vi "Methods_Insert Dividers.vi"(11 "Methods[] In":T1(array[cluster])) -> (3 "Methods[] Out":T1(array[cluster]))   [LabVIEW 2023] (continued)
"Data name"="Statechart.Open Private", "Short name (localized)"="Statechart.Open Private", "Long name (localized)"="Statechart:Open Private"}, "Method Flags"={"IsDeprecated"=FALSE, "IsPrivate"=TRUE, "IsScripting"=FALSE, "IsNotInRun-Time"=FALSE}, "Divider"=FALSE}, {"Class Info"={"Unique ID string"="1", "Parent ID string"="", "Class Name (unlocalized)"="Application", "Class Name (localized)"="Application"}, "Method Info"={"Unique ID string"="90f", "Data name"="Project.DoingAutosaveRecovery", "Short name (localized)"="Project.DoingAutosaveRecovery", "Long name (localized)"="Project:Doing Auto Save Recovery"}, "Method Flags"={"IsDeprecated"=FALSE, "IsPrivate"=TRUE, "IsScripting"=FALSE, "IsNotInRun-Time"=FALSE}, "Divider"=FALSE}, {"Class Info"={"Unique ID string"="1", "Parent ID string"="", "Class Name (unlocalized)"="Application", "Class Name (localized)"="Application"}, "Method Info"={"Unique ID string"="910", "Data name"="AllowScripting", "Short name (localized)"="AllowScripting", "Long name (localized)"="Allow Scripting"}, "Method Flags"={"IsDeprecated"=FALSE, "IsPrivate"=TRUE, "IsScripting"=TRUE, "IsNotInRun-Time"=FALSE}, "Divider"=FALSE}, {"Class Info"={"Unique ID string"="1", "Parent ID string"="", "Class Name (unlocalized)"="Application", "Class Name (localized)"="Application"}, "Method Info"={"Unique ID string"="911", "Data name"="EnableExternalProptypes", "Short name (localized)"="EnableExternalProptypes", "Long name (localized)"="Enable External Proptypes"}, "Method Flags"={"IsDeprecated"=FALSE, "IsPrivate"=TRUE, "IsScripting"=TRUE, "IsNotInRun-Time"=FALSE}, "Divider"=FALSE}, {"Class Info"={"Unique ID string"="1", "Parent ID string"="", "Class Name (unlocalized)"="Application", "Class Name (localized)"="Application"}, "Method Info"={"Unique ID string"="912", "Data name"="EnableTempSelect", "Short name (localized)"="EnableTempSelect", "Long name (localized)"="Enable Temp Selection"}, "Method Flags"={"IsDeprecated"=FALSE, "IsPrivate"=TRUE, "IsScripting"=FALSE, "IsNotInRun-Time"=FALSE}, "Divider"=FALSE}, {"Class Info"={"Unique ID string"="1", "Parent ID string"="", "Class Name (unlocalized)"="Application", "Class Name (localized)"="Application"}, "Method Info"={"Unique ID string"="913", "Data name"="EnableMetaTrans", "Short name (localized)"="EnableMetaTrans", "Long name (localized)"="Enable Meta Transactions"}, "Method Flags"={"IsDeprecated"=FALSE, "IsPrivate"=TRUE, "IsScripting"=TRUE, "IsNotInRun-Time"=FALSE}, "Divider"=FALSE}, {"Class Info"={"Unique ID string"="1", "Parent ID string"="", "Class Name (unlocalized)"="Application", "Class Name (localized)"="Application"}, "Method Info"={"Unique ID string"="914", "Data name"="Symbols.GetValue", "Short name (localized)"="Symbols.GetValue", "Long name (localized)"="Symbols:Get Value"}, "Method Flags"={"IsDeprecated"=FALSE, "IsPrivate"=TRUE, "IsScripting"=FALSE, "IsNotInRun-Time"=TRUE}, "Divider"=FALSE}, {"Class Info"={"Unique ID string"="1", "Parent ID string"="", "Class Name (unlocalized)"="Application", "Class Name (localized)"="Application"}, "Method Info"={"Unique ID string"="915", "Data name"="DeferErrWinUpdates", "Short name (localized)"="DeferErrWinUpdates", "Long name (localized)"="Error Window:Defer Updates"}, "Method Flags"={"IsDeprecated"=FALSE, "IsPrivate"=TRUE, "IsScripting"=FALSE, "IsNotInRun-Time"=TRUE}, "Divider"=FALSE}, {"Class Info"={"Unique ID string"="1", "Parent ID string"="", "Class Name (unlocalized)"="Application", "Class Name (localized)"="Application"}, "Method Info"={"Unique ID string"="916", "Data name"="DTT.IsTracingEnabled", "Short name (localized)"="DTT.IsTracingEnabled", "Long name (localized)"="Desktop Tracing:Is Tracing Enabled"}, "Method Flags"={"IsDeprecated"=FALSE, "IsPrivate"=TRUE, "IsScripting"=FALSE, "IsNotInRun-Time"=FALSE}, "Divider"=FALSE}, {"Class Info"={"Unique ID string"="1", "Parent ID string"="", "Class Name (unlocalized)"="Application", "Class Name (localized)"="Application"}, "Method Info"={"Unique ID string"="917", "Data name"="WebSrvr.Conf", "Short name (localized)"="WebSrvr.Conf", "Long name (localized)"="Web Server:Configure"}, "Method Flags"={"IsDeprecated"=FALSE, "IsPrivate"=FALSE, "IsScripting"=FALSE, "IsNotInRun-Time"=FALSE}, "Divider"=FALSE}, {"Class Info"={"Unique ID string"="1", "Parent ID string"="", "Class Name (unlocalized)"="Application", "Class Name (localized)"="Application"}, "Method Info"={"Unique ID string"="918", "Data name"="CheckMathScriptWatchedPaths", "Short name (localized)"="CheckMathScriptWatchedPaths", "Long name (localized)"="MathScript:Check Watched Paths"}, "Method Flags"={"IsDeprecated"=FALSE, "IsPrivate"=TRUE, "IsScripting"=TRUE, "IsNotInRun-Time"=TRUE}, "Divider"=FALSE}, {"Class Info"={"Unique ID string"="1", "Parent ID string"="", "Class Name (unlocalized)"="Application", "Class Name (localized)"="Application"}, "Method Info"={"Unique ID string"="919", "Data name"="Open.LV Documents", "Short name (localized)"="Open.LV Documents", "Long name (localized)"="Open:LabVIEW Documents"}, "Method Flags"={"IsDeprecated"=FALSE, "IsPrivate"=TRUE, "IsScripting"=FALSE, "IsNotInRun-Time"=TRUE}, "Divider"=FALSE}, {"Class Info"={"Unique ID string"="1", "Parent ID string"="", "Class Name (unlocalized)"="Application", "Class Name (localized)"="Application"}, "Method Info"={"Unique ID string"="91a", "Data name"="Get VI.ConPane DataType", "Short name (localized)"="Get VI.ConPane DataType", "Long name (localized)"="Get VI:ConPane DataType"}, "Method Flags"={"IsDeprecated"=FALSE, "IsPrivate"=FALSE, "IsScripting"=TRUE, "IsNotInRun-Time"=FALSE}, "Divider"=FALSE}, {"Class Info"={"Unique ID string"="1", "Parent ID string"="", "Class Name (unlocalized)"="Application", "Class Name (localized)"="Application"}, "Method Info"={"Unique ID string"="91b", "Data name"="GetActiveVIRef", "Short name (localized)"="GetActiveVIRef", "Long name (localized)"="Get Active VI Reference"}, "Method Flags"={"IsDeprecated"=FALSE, "IsPrivate"=FALSE, "IsScripting"=TRUE, "IsNotInRun-Time"=TRUE}, "Divider"=FALSE}, {"Class Info"={"Unique ID string"="1", "Parent ID string"="", "Class Name (unlocalized)"="Application", "Class Name (localized)"="Application"}, "Method Info"={"Unique ID string"="91c", "Data name"="CodeCov.Start", "Short name (localized)"="CodeCov.Start", "Long name (localized)"="Code Coverage:Start"}, "Method Flags"={"IsDeprecated"=FALSE, "IsPrivate"=TRUE, "IsScripting"=FALSE, "IsNotInRun-Time"=TRUE}, "Divider"=FALSE}, {"Class Info"={"Unique ID string"="1", "Parent ID string"="", "Class Name (unlocalized)"="Application", "Class Name (localized)"="Application"}, "Method Info"={"Unique ID string"="91d", "Data name"="CodeCov.Stop", "Short name (localized)"="CodeCov.Stop", "Long name (localized)"="Code Coverage:Stop"}, "Method Flags"={"IsDeprecated"=FALSE, "IsPrivate"=TRUE, "IsScripting"=FALSE, "IsNotInRun-Time"=TRUE}, "Divider"=FALSE}, {"Class Info"={"Unique ID string"="1", "Parent ID string"="", "Class Name (unlocalized)"="Application", "Class Name (localized)"="Application"}, "Method Info"={"Unique ID string"="91e", "Data name"="CodeCov.Reset", "Short name (localized)"="CodeCov.Reset", "Long name (localized)"="Code Coverage:Reset"}, "Method Flags"={"IsDeprecated"=FALSE, "IsPrivate"=TRUE, "IsScripting"=FALSE, "IsNotInRun-Time"=TRUE}, "Divider"=FALSE}, {"Class Info"={"Unique ID string"="1", "Parent ID string"="", "Class Name (unlocalized)"="Application", "Class Name (localized)"="Application"}, "Method Info"={"Unique ID string"="91f", "Data name"="CodeCov.Reset VI", "Short name (localized)"="CodeCov.Reset VI", "Long name (localized)"="Code Coverage:Reset VI"}, "Method Flags"={"IsDeprecated"=FALSE, "IsPrivate"=TRUE, "IsScripting"=FALSE, "IsNotInRun-Time"=TRUE}, "Divider"=FALSE}, {"Class Info"={"Unique ID string"="1", "Parent ID string"="", "Class Name (unlocalized)"="Application", "Class Name (localized)"="Application"}, "Method Info"={"Unique ID string"="920", "Data name"="CodeCov.AllVIs", "Short name (localized)"="CodeCov.AllVIs", "Long name (localized)"="Code Coverage:All VIs Measured"}, "Method Flags"={"IsDeprecated"=FALSE, "IsPrivate"=TRUE, "IsScripting"=FALSE, "IsNotInRun-Time"=TRUE}, "Divider"=FALSE}, {"Class Info"={"Unique ID string"="1", "Parent ID string"="", "Class Name (unlocalized)"="Application", "Class Name (localized)"="Application"}, "Method Info"={"Unique ID string"="921", "Data name"="CodeCov.VIPercentage", "Short name (localized)"="CodeCov.VIPercentage", "Long name (localized)"="Code Coverage:VI Percentage"}, "Method Flags"={"IsDeprecated"=FALSE, "IsPrivate"=TRUE, "IsScripting"=FALSE, "IsNotInRun-Time"=TRUE}, "Divider"=FALSE}, {"Class Info"={"Unique ID string"="1", "Parent ID string"="", "Class Name (unlocalized)"="Application", "Class Name (localized)"="Application"}, "Method Info"={"Unique ID string"="922", "Data name"="CodeCov.UnrunDiags", "Short name (localized)"="CodeCov.UnrunDiags", "Long name (localized)"="Code Coverage:Uncovered Diagrams"}, "Method Flags"={"IsDeprecated"=FALSE, "IsPrivate"=TRUE, "IsScripting"=FALSE, "IsNotInRun-Time"=TRUE}, "Divider"=FALSE}, {"Class Info"={"Unique ID string"="1", "Parent ID string"="", "Class Name (unlocalized)"="Application", "Class Name (localized)"="Application"}, "Method Info"={"Unique ID string"="923", "Data name"="CodeCov.ShowUnrunDiags", "Short name (localized)"="CodeCov.ShowUnrunDiags", "Long name (localized)"="Code Coverage:Show Uncovered Diagrams"}, "Method Flags"={"IsDeprecated"=FALSE, "IsPrivate"=TRUE, "IsScripting"=FALSE, "IsNotInRun-Time"=TRUE}, "Divider"=FALSE}, {"Class Info"={"Unique ID string"="1", "Parent ID string"="", "Class Name (unlocalized)"="Application", "Class Name (localized)"="Application"}, "Method Info"={"Unique ID string"="924", "Data name"="UI:Abort Merge VIs", "Short name (localized)"="UI:Abort Merge VIs", "Long name (localized)"="User Interaction:Abort Merge VIs"}, "Method Flags"={"IsDeprecated"=FALSE, "IsPrivate"=TRUE, "IsScripting"=FALSE, "IsNotInRun-Time"=TRUE}, "Divider"=FALSE}, {"Class Info"={"Unique ID string"="1", "Parent ID string"="", "Class Name (unlocalized)"="Application", "Class Name (localized)"="Application"}, "Method Info"={"Unique ID string"="925", "Data name"="UI:Merge Load VI", "Short name (localized)"="UI:Merge Load VI", "Long name (localized)"="User Interaction:Merge Load VI"}, "Method Flags"={"IsDeprecated"=FALSE, "IsPrivate"=TRUE, "IsScripting"=FALSE, "IsNotInRun-Time"=TRUE}, "Divider"=FALSE}, {"Class Info"={"Unique ID string"="1", "Parent ID string"="", "Class Name (unlocalized)"="Application", "Class Name (localized)"="Application"}, "Method Info"={"Unique ID string"="926", "Data name"="UI:Merge Save VI", "Short name (localized)"="UI:Merge Save VI", "Long name (localized)"="User Interaction:Merge Save VI"}, "Method Flags"={"IsDeprecated"=FALSE, "IsPrivate"=TRUE, "IsScripting"=FALSE, "IsNotInRun-Time"=TRUE}, "Divider"=FALSE}, {"Class Info"={"Unique ID string"="1", "Parent ID string"="", "Class Name (unlocalized)"="Application", "Class Name (localized)"="Application"}, "Method Info"={"Unique ID string"="927", "Data name"="UI:Merge Cross Load VI", "Short name (localized)"="UI:Merge Cross Load VI", "Long name (localized)"="User Interaction:Merge Cross Load VI"}, "Method Flags"={"IsDeprecated"=FALSE, "IsPrivate"=TRUE, "IsScripting"=FALSE, "IsNotInRun-Time"=TRUE}, "Divider"=FALSE}, {"Class Info"={"Unique ID string"="1", "Parent ID string"="", "Class Name (unlocalized)"="Application", "Class Name (localized)"="Application"}, "Method Info"={"Unique ID string"="928", "Data name"="UI:Merge Close VI", "Short name (localized)"="UI:Merge Close VI", "Long name (localized)"="User Interaction:Merge Close VI"}, "Method Flags"={"IsDeprecated"=FALSE, "IsPrivate"=TRUE, "IsScripting"=FALSE, "IsNotInRun-Time"=TRUE}, "Divider"=FALSE}, {"Class Info"={"Unique ID string"="1", "Parent ID string"="", "Class Name (unlocalized)"="Application", "Class Name (localized)"="Application"}, "Method Info"={"Unique ID string"="929", "Data name"="UI:Merge Load Library", "Short name (localized)"="UI:Merge Load Library", "Long name (localized)"="User Interaction:Merge Load Library"}, "Method Flags"={"IsDeprecated"=FALSE, "IsPrivate"=TRUE, "IsScripting"=FALSE, "IsNotInRun-Time"=TRUE}, "Divider"=FALSE}, {"Class Info"={"Unique ID string"="1", "Parent ID string"="", "Class Name (unlocalized)"="Application", "Class Name (localized)"="Application"}, "Method Info"={"Unique ID string"="92a", "Data name"="UI:Merge Close Library", "Short name (localized)"="UI:Merge Close Library", "Long name (localized)"="User Interaction:Merge Close Library"}, "Method Flags"={"IsDeprecated"=FALSE, "IsPrivate"=TRUE, "IsScripting"=FALSE, "IsNotInRun-Time"=TRUE}, "Divider"=FALSE}, {"Class Info"={"Unique ID string"="1", "Parent ID string"="", "Class Name (unlocalized)"="Application", "Class Name (localized)"="Application"}, "Method Info"={"Unique ID string"="92b", "Data name"="UI:Merge Clean Up Context", "Short name (localized)"="UI:Merge Clean Up Context", "Long name (localized)"="User Interaction:Merge Clean Up Context"}, "Method Flags"={"IsDeprecated"=FALSE, "IsPrivate"=TRUE, "IsScripting"=FALSE, "IsNotInRun-Time"=TRUE}, "Divider"=FALSE}, {"Class Info"={"Unique ID string"="1", "Parent ID string"="", "Class Name (unlocalized)"="Application", "Class Name (localized)"="Application"}, "Method Info"={"Unique ID string"="92c", "Data name"="UI:Merge Save Library", "Short name (localized)"="UI:Merge Save Library", "Long name (localized)"="User Interaction:Merge Save Library"}, "Method Flags"={"IsDeprecated"=FALSE, "IsPrivate"=TRUE, "IsScripting"=FALSE, "IsNotInRun-Time"=TRUE}, "Divider"=FALSE}, {"Class Info"={"Unique ID string"="1", "Parent ID string"="", "Class Name (unlocalized)"="Application", "Class Name (localized)"="Application"}, "Method Info"={"Unique ID string"="92d", "Data name"="License.Get Feature Activators", "Short name (localized)"="License.Get Feature Activators", "Long name (localized)"="License:Get Feature Activators"}, "Method Flags"={"IsDeprecated"=FALSE, "IsPrivate"=TRUE, "IsScripting"=FALSE, "IsNotInRun-Time"=FALSE}, "Divider"=FALSE}, {"Class Info"={"Unique ID string"="1", "Parent ID string"="", "Class Name (unlocalized)"="Application", "Class Name (localized)"="Application"}, "Method Info"={"Unique ID string"="92e", "Data name"="UI:Merge Load Refees", "Short name (localized)"="UI:Merge Load Refees", "Long name (localized)"="User Interaction:Merge Load Refees"}, "Method Flags"={"IsDeprecated"=FALSE, "IsPrivate"=TRUE, "IsScripting"=FALSE, "IsNotInRun-Time"=TRUE}, "Divider"=FALSE}, {"Class Info"={"Unique ID string"="1", "Parent ID string"="", "Class Name (unlocalized)"="Application", "Class Name (localized)"="Application"}, "Method Info"={"Unique ID string"="92f", "Data name"="Library.Undeploy Libraries", "Short name (localized)"="Library.Undeploy Libraries", "Long name (localized)"="Library:Undeploy Libraries"}, "Method Flags"={"IsDeprecated"=FALSE, "IsPrivate"=FALSE, "IsScripting"=FALSE, "IsNotInRun-Time"=FALSE}, "Divider"=FALSE}, {"Class Info"={"Unique ID string"="1", "Parent ID string"="", "Class Name (unlocalized)"="Application", "Class Name (localized)"="Application"}, "Method Info"={"Unique ID string"="930", "Data name"="Close All Palettes", "Short name (localized)"="Close All Palettes", "Long name (localized)"="Palettes:Close All Palettes"}, "Method Flags"={"IsDeprecated"=FALSE, "IsPrivate"=FALSE, "IsScripting"=FALSE, "IsNotInRun-Time"=TRUE}, "Divider"=FALSE}, {"Class Info"={"Unique ID string"="1", "Parent ID string"="", "Class Name (unlocalized)"="Application", "Class Name (localized)"="Application"}, "Method Info"={"Unique ID string"="931", "Data name"="UI.Edit Icon", "Short name (localized)"="UI.Edit Icon", "Long name (localized)"="User Interaction:Edit Icon"}, "Method Flags"={"IsDeprecated"=FALSE, "IsPrivate"=TRUE, "IsScripting"=FALSE, "IsNotInRun-Time"=TRUE}, "Divider"=FALSE}, {"Class Info"={"Unique ID string"="1", "Parent ID string"="", "Class Name (unlocalized)"="Application", "Class Name (localized)"="Application"}, "Method Info"={"Unique ID string"="932", "Data name"="CreateInstantiation", "Short name (localized)"="CreateInstantiation", "Long name (localized)"="Create Generic VI Instantiation"}, "Method Flags"={"IsDeprecated"=FALSE, "IsPrivate"=TRUE, "IsScripting"=TRUE, "IsNotInRun-Time"=TRUE}, "Divider"=FALSE}, {"Class Info"={"Unique ID string"="1", "Parent ID string"="", "Class Name (unlocalized)"="Application", "Class Name (localized)"="Application"}, "Method Info"={"Unique ID string"="933", "Data name"="Move VIs", "Short name (localized)"="Move VIs", "Long name (localized)"="Move VIs"}, "Method Flags"={"IsDeprecated"=FALSE, "IsPrivate"=TRUE, "IsScripting"=FALSE, "IsNotInRun-Time"=FALSE}, "Divider"=FALSE}, {"Class Info"={"Unique ID string"="1", "Parent ID string"="", "Class Name (unlocalized)"="Application", "Class Name (localized)"="Application"}, "Method Info"={"Unique ID string"="935", "Data name"="Library.Get Ref By Qualified Name", "Short name (localized)"="Library.Get Ref By Qualified Name", "Long name (localized)"="Library:Get Ref By Qualified Name"}, "Method Flags"={"IsDeprecated"=FALSE, "IsPrivate"=FALSE, "IsScripting"=FALSE, "IsNotInRun-Time"=FALSE}, "Divider"=FALSE}, {"Class Info"={"Unique ID string"="1", "Parent ID string"="", "Class Name (unlocalized)"="Application", "Class Name (localized)"="Application"}, "Method Info"={"Unique ID string"="936", "Data name"="CopyDataConvert", "Short name (localized)"="CopyDataConvert", "Long name (localized)"="Copy Data Convert"}, "Method Flags"={"IsDeprecated"=FALSE, "IsPrivate"=TRUE, "IsScripting"=TRUE, "IsNotInRun-Time"=FALSE}, "Divider"=FALSE}, {"Class Info"={"Unique ID string"="1", "Parent ID string"="", "Class Name (unlocalized)"="Application", "Class Name (localized)"="Application"}, "Method Info"={"Unique ID string"="937", "Data name"="LoadMSCompiler", "Short name (localized)"="LoadMSCompiler", "Long name (localized)"="MathScript:Load MathScript Compiler"}, "Method Flags"={"IsDeprecated"=FALSE, "IsPrivate"=TRUE, "IsScripting"=FALSE, "IsNotInRun-Time"=TRUE}, "Divider"=FALSE}, {"Class Info"={"Unique ID string"="1", "Parent ID string"="", "Class Name (unlocalized)"="Application", "Class Name (localized)"="Application"}, "Method Info"={"Unique ID string"="938", "Data name"="Get Hier Img Scaled", "Short name (localized)"="Get Hier Img Scaled", "Long name (localized)"="Get VI Hierarchy Image Scaled"}, "Method Flags"={"IsDeprecated"=FALSE, "IsPrivate"=FALSE, "IsScripting"=FALSE, "IsNotInRun-Time"=FALSE}, "Divider"=FALSE}, {"Class Info"={"Unique ID string"="1", "Parent ID string"="", "Class Name (unlocalized)"="Application", "Class Name (localized)"="Application"}, "Method Info"={"Unique ID string"="939", "Data name"="SearchOpenSession", "Short name (localized)"="SearchOpenSession", "Long name (localized)"="Search:Open Session"}, "Method Flags"={"IsDeprecated"=FALSE, "IsPrivate"=TRUE, "IsScripting"=FALSE, "IsNotInRun-Time"=TRUE}, "Divider"=FALSE}, {"Class Info"={"Unique ID string"="1", "Parent ID string"="", "Class Name (unlocalized)"="Application", "Class Name (localized)"="Application"}, "Method Info"={"Unique ID string"="93a", "Data name"="SearchCloseSession", "Short name (localized)"="SearchCloseSession", "Long name (localized)"="Search:Close Session"}, "Method Flags"={"IsDeprecated"=FALSE, "IsPrivate"=TRUE, "IsScripting"=FALSE, "IsNotInRun-Time"=TRUE}, "Divider"=FALSE}, {"Class Info"={"Unique ID string"="1", "Parent ID string"="", "Class Name (unlocalized)"="Application", "Class Name (localized)"="Application"}, "Method Info"={"Unique ID string"="93b", "Data name"="SearchLoadPlugin", "Short name (localized)"="SearchLoadPlugin", "Long name (localized)"="Search:Load Plugin"}, "Method Flags"={"IsDeprecated"=FALSE, "IsPrivate"=TRUE, "IsScripting"=FALSE, "IsNotInRun-Time"=TRUE}, "Divider"=FALSE}, {"Class Info"={"Unique ID string"="1", "Parent ID string"="", "Class Name (unlocalized)"="Application", "Class Name (localized)"="Application"}, "Method Info"={"Unique ID string"="93c", "Data name"="SearchInitSession", "Short name (localized)"="SearchInitSession", "Long name (localized)"="Search:Init Session"}, "Method Flags"={"IsDeprecated"=FALSE, "IsPrivate"=TRUE, "IsScripting"=FALSE, "IsNotInRun-Time"=TRUE}, "Divider"=FALSE}, {"Class Info"={"Unique ID string"="1", "Parent ID string"="", "Class Name (unlocalized)"="Application", "Class Name (localized)"="Application"}, "Method Info"={"Unique ID string"="93d", "Data name"="SearchSyncSearch", "Short name (localized)"="SearchSyncSearch", "Long name (localized)"="Search:SyncSearch"}, "Method Flags"={"IsDeprecated"=FALSE, "IsPrivate"=TRUE, "IsScripting"=FALSE, "IsNotInRun-Time"=TRUE}, "Divider"=FALSE}, {"Class Info"={"Unique ID string"="1", "Parent ID string"="", "Class Name (unlocalized)"="Application", "Class Name (localized)"="Application"}, "Method Info"={"Unique ID string"="93e", "Data name"="SearchSyncSearchForQD", "Short name (localized)"="SearchSyncSearchForQD", "Long name (localized)"="Search:Sync Search For QD"}, "Method Flags"={"IsDeprecated"=FALSE, "IsPrivate"=TRUE, "IsScripting"=FALSE, "IsNotInRun-Time"=TRUE}, "Divider"=FALSE}, {"Class Info"={"Unique ID string"="1", "Parent ID string"="", "Class Name (unlocalized)"="Application", "Class Name (localized)"="Application"}, "Method Info"={"Unique ID string"="93f", "Data name"="UI.PlaceObjectOnCursor", "Short name (localized)"="UI.PlaceObjectOnCursor", "Long name (localized)"="User Interaction:Place Object On Cursor"}, "Method Flags"={"IsDeprecated"=FALSE, "IsPrivate"=FALSE, "IsScripting"=TRUE, "IsNotInRun-Time"=TRUE}, "Divider"=FALSE}, {"Class Info"={"Unique ID string"="1", "Parent ID string"="", "Class Name (unlocalized)"="Application", "Class Name (localized)"="Application"}, "Method Info"={"Unique ID string"="940", "Data name"="UI.Drop Proj Item Copy", "Short name (localized)"="UI.Drop Proj Item Copy", "Long name (localized)"="User Interaction:Place Project Item On Cursor"}, "Method Flags"={"IsDeprecated"=FALSE, "IsPrivate"=TRUE, "IsScripting"=FALSE, "IsNotInRun-Time"=TRUE}, "Divider"=FALSE}, {"Class Info"={"Unique ID string"="1", "Parent ID string"="", "Class Name (unlocalized)"="Application", "Class Name (localized)"="Application"}, "Method Info"={"Unique ID string"="941", "Data name"="UpdateNXTContextName", "Short name (localized)"="UpdateNXTContextName", "Long name (localized)"="NXT:Update Context Name"}, "Method Flags"={"IsDeprecated"=FALSE, "IsPrivate"=TRUE, "IsScripting"=FALSE, "IsNotInRun-Time"=TRUE}, "Divider"=FALSE}, {"Class Info"={"Unique ID string"="1", "Parent ID string"="", "Class Name (unlocalized)"="Application", "Class Name (localized)"="Application"}, "Method Info"={"Unique ID string"="942", "Data name"="ClearInstantiationCacheCache", "Short name (localized)"="ClearInstantiationCacheCache", "Long name (localized)"="Clear Instantiation Cache Cache"}, "Method Flags"={"IsDeprecated"=FALSE, "IsPrivate"=TRUE, "IsScripting"=FALSE, "IsNotInRun-Time"=TRUE}, "Divider"=FALSE}, {"Class Info"={"Unique ID string"="1", "Parent ID string"="", "Class Name (unlocalized)"="Application", "Class Name (localized)"="Application"}, "Method Info"={"Unique ID string"="943", "Data name"="GetInstantiationConPaneFromCache", "Short name (localized)"="GetInstantiationConPaneFromCache", "Long name (localized)"="Get Instantiation ConPane From Cache"}, "Method Flags"={"IsDeprecated"=FALSE, "IsPrivate"=TRUE, "IsScripting"=FALSE, "IsNotInRun-Time"=TRUE}, "Divider"=FALSE}, {"Class Info"={"Unique ID string"="1", "Parent ID string"="", "Class Name (unlocalized)"="Application", "Class Name (localized)"="Application"}, "Method Info"={"Unique ID string"="944", "Data name"="DTT.FilterVILibEvents", "Short name (localized)"="DTT.FilterVILibEvents", "Long name (localized)"="Desktop Tracing:Filter VI Lib Events"}, "Method Flags"={"IsDeprecated"=FALSE, "IsPrivate"=TRUE, "IsScripting"=FALSE, "IsNotInRun-Time"=FALSE}, "Divider"=FALSE}, {"Class Info"={"Unique ID string"="1", "Parent ID string"="", "Class Name (unlocalized)"="Application", "Class Name (localized)"="Application"}, "Method Info"={"Unique ID string"="945", "Data name"="LocateMSTargetSyntaxVI", "Short name (localized)"="LocateMSTargetSyntaxVI", "Long name (localized)"="MathScript:Locate Math Script Target Syntax VI"}, "Method Flags"={"IsDeprecated"=FALSE, "IsPrivate"=TRUE, "IsScripting"=FALSE, "IsNotInRun-Time"=TRUE}, "Divider"=FALSE}, {"Class Info"={"Unique ID string"="1", "Parent ID string"="", "Class Name (unlocalized)"="Application", "Class Name (localized)"="Application"}, "Method Info"={"Unique ID string"="946", "Data name"="GetEnvModePath", "Short name (localized)"="GetEnvModePath", "Long name (localized)"="Get Environment Mode Settings Path"}, "Method Flags"={"IsDeprecated"=FALSE, "IsPrivate"=TRUE, "IsScripting"=FALSE, "IsNotInRun-Time"=TRUE}, "Divider"=FALSE}, {"Class Info"={"Unique ID string"="1", "Parent ID string"="", "Class Name (unlocalized)"="Application", "Class Name (localized)"="Application"}, "Method Info"={"Unique ID string"="947", "Data name"="Get VI Editor Version", "Short name (localized)"="Get VI Editor Version", "Long name (localized)"="Get VI:Editor Version"}, "Method Flags"={"IsDeprecated"=FALSE, "IsPrivate"=FALSE, "IsScripting"=FALSE, "IsNotInRun-Time"=FALSE}, "Divider"=FALSE}, {"Class Info"={"Unique ID string"="1", "Parent ID string"="", "Class Name (unlocalized)"="Application", "Class Name (localized)"="Application"}, "Method Info"={"Unique ID string"="948", "Data name"="Get VI.Qualified Name", "Short name (localized)"="Get VI.Qualified Name", "Long name (localized)"="Get VI:Qualified Name"}, "Method Flags"={"IsDeprecated"=FALSE, "IsPrivate"=FALSE, "IsScripting"=FALSE, "IsNotInRun-Time"=FALSE}, "Divider"=FALSE}, {"Class Info"={"Unique ID string"="1", "Parent ID string"="", "Class Name (unlocalized)"="Application", "Class Name (localized)"="Application"}, "Method Info"={"Unique ID string"="949", "Data name"="OpenVIInNXTContext", "Short name (localized)"="OpenVIInNXTContext", "Long name (localized)"="NXT:Open VI In Context"}, "Method Flags"={"IsDeprecated"=FALSE, "IsPrivate"=TRUE, "IsScripting"=FALSE, "IsNotInRun-Time"=TRUE}, "Divider"=FALSE}, {"Class Info"={"Unique ID string"="1", "Parent ID string"="", "Class Name (unlocalized)"="Application", "Class Name (localized)"="Application"}, "Method Info"={"Unique ID string"="94b", "Data name"="App.PrepareToLoadFiles", "Short name (localized)"="App.PrepareToLoadFiles", "Long name (localized)"="Prepare to Load Files"}, "Method Flags"={"IsDeprecated"=FALSE, "IsPrivate"=TRUE, "IsScripting"=FALSE, "IsNotInRun-Time"=FALSE}, "Divider"=FALSE}, {"Class Info"={"Unique ID string"="1", "Parent ID string"="", "Class Name (unlocalized)"="Application", "Class Name (localized)"="Application"}, "Method Info"={"Unique ID string"="94c", "Data name"="Get Pal Item Icon", "Short name (localized)"="Get Pal Item Icon", "Long name (localized)"="Palettes:Get Palette Item Icon"}, "Method Flags"={"IsDeprecated"=FALSE, "IsPrivate"=TRUE, "IsScripting"=FALSE, "IsNotInRun-Time"=TRUE}, "Divider"=FALSE}, {"Class Info"={"Unique ID string"="1", "Parent ID string"="", "Class Name (unlocalized)"="Application", "Class Name (localized)"="Application"}, "Method Info"={"Unique ID string"="94d", "Data name"="ReadDFIRTokens", "Short name (localized)"="ReadDFIRTokens", "Long name (localized)"="Compiler:Read DFIR Tokens"}, "Method Flags"={"IsDeprecated"=FALSE, "IsPrivate"=TRUE, "IsScripting"=FALSE, "IsNotInRun-Time"=FALSE}, "Divider"=FALSE}, {"Class Info"={"Unique ID string"="1", "Parent ID string"="", "Class Name (unlocalized)"="Application", "Class Name (localized)"="Application"}, "Method Info"={"Unique ID string"="94e", "Data name"="CreateProbeVIFromVariant", "Short name (localized)"="CreateProbeVIFromVariant", "Long name (localized)"="Probes:Create Probe VI From Variant"}, "Method Flags"={"IsDeprecated"=FALSE, "IsPrivate"=TRUE, "IsScripting"=TRUE, "IsNotInRun-Time"=TRUE}, "Divider"=FALSE}, {"Class Info"={"Unique ID string"="1", "Parent ID string"="", "Class Name (unlocalized)"="Application", "Class Name (localized)"="Application"}, "Method Info"={"Unique ID string"="94f", "Data name"="GetProbePathListFromVariant", "Short name (localized)"="GetProbePathListFromVariant", "Long name (localized)"="Probes:Get Probe Path List From Variant"}, "Method Flags"={"IsDeprecated"=FALSE, "IsPrivate"=TRUE, "IsScripting"=TRUE, "IsNotInRun-Time"=TRUE}, "Divider"=FALSE}, {"Class Info"={"Unique ID string"="1", "Parent ID string"="", "Class Name (unlocalized)"="Application", "Class Name (localized)"="Application"}, "Method Info"={"Unique ID string"="951", "Data name"="Build.PackedLibrary", "Short name (localized)"="Build.PackedLibrary", "Long name (localized)"="Build:PackedLibrary"}, "Method Flags"={"IsDeprecated"=FALSE, "IsPrivate"=TRUE, "IsScripting"=FALSE, "IsNotInRun-Time"=TRUE}, "Divider"=FALSE}, {"Class Info"={"Unique ID string"="1", "Parent ID string"="", "Class Name (unlocalized)"="Application", "Class Name (localized)"="Application"}, "Method Info"={"Unique ID string"="952", "Data name"="GetCompilerSettings", "Short name (localized)"="GetCompilerSettings", "Long name (localized)"="Compiler:Get Compiler Settings"}, "Method Flags"={"IsDeprecated"=FALSE, "IsPrivate"=TRUE, "IsScripting"=FALSE, "IsNotInRun-Time"=FALSE}, "Divider"=FALSE}, {"Class Info"={"Unique ID string"="1", "Parent ID string"="", "Class Name (unlocalized)"="Application", "Class Name (localized)"="Application"}, "Method Info"={"Unique ID string"="953", "Data name"="SetCompilerSettings", "Short name (localized)"="SetCompilerSettings", "Long name (localized)"="Compiler:Set Compiler Settings"}, "Method Flags"={"IsDeprecated"=FALSE, "IsPrivate"=TRUE, "IsScripting"=FALSE, "IsNotInRun-Time"=FALSE}, "Divider"=FALSE}, {"Class Info"={"Unique ID string"="1", "Parent ID string"="", "Class Name (unlocalized)"="Application", "Class Name (localized)"="Application"}, "Method Info"={"Unique ID string"="954", "Data name"="Project.GetFileLVVersion", "Short name (localized)"="Project.GetFileLVVersion", "Long name (localized)"="Project:Get File LabVIEW Version"}, "Method Flags"={"IsDeprecated"=FALSE, "IsPrivate"=FALSE, "IsScripting"=FALSE, "IsNotInRun-Time"=FALSE}, "Divider"=FALSE}, {"Class Info"={"Unique ID string"="1", "Parent ID string"="", "Class Name (unlocalized)"="Application", "Class Name (localized)"="Application"}, "Method Info"={"Unique ID string"="955", "Data name"="Save All", "Short name (localized)"="Save All", "Long name (localized)"="Save All"}, "Method Flags"={"IsDeprecated"=FALSE, "IsPrivate"=TRUE, "IsScripting"=FALSE, "IsNotInRun-Time"=FALSE}, "Divider"=FALSE}, {"Class Info"={"Unique ID string"="1", "Parent ID string"="", "Class Name (unlocalized)"="Application", "Class Name (localized)"="Application"}, "Method Info"={"Unique ID string"="956", "Data name"="Release LV Class Cookies", "Short name (localized)"="Release LV Class Cookies", "Long name (localized)"="LabVIEW Class:Release LV Class Cookies"}, "Method Flags"={"IsDeprecated"=FALSE, "IsPrivate"=TRUE, "IsScripting"=FALSE, "IsNotInRun-Time"=FALSE}, "Divider"=FALSE}, {"Class Info"={"Unique ID string"="1", "Parent ID string"="", "Class Name (unlocalized)"="Application", "Class Name (localized)"="Application"}, "Method Info"={"Unique ID string"="957", "Data name"="Consolidated Save", "Short name (localized)"="Consolidated Save", "Long name (localized)"="Consolidated Save"}, "Method Flags"={"IsDeprecated"=FALSE, "IsPrivate"=TRUE, "IsScripting"=FALSE, "IsNotInRun-Time"=TRUE}, "Divider"=FALSE}, {"Class Info"={"Unique ID string"="1", "Parent ID string"="", "Class Name (unlocalized)"="Application", "Class Name (localized)"="Application"}, "Method Info"={"Unique ID string"="958", "Data name"="Compare CPTMs For Packed Library", "Short name (localized)"="Compare CPTMs For Packed Library", "Long name (localized)"="Compare:CPTMs For Packed Library"}, "Method Flags"={"IsDeprecated"=FALSE, "IsPrivate"=TRUE, "IsScripting"=FALSE, "IsNotInRun-Time"=FALSE}, "Divider"=FALSE}, {"Class Info"={"Unique ID string"="1", "Parent ID string"="", "Class Name (unlocalized)"="Application", "Class Name (localized)"="Application"}, "Method Info"={"Unique ID string"="959", "Data name"="Get Pal Item Path", "Short name (localized)"="Get Pal Item Path", "Long name (localized)"="Palettes:Get Palette Item Path"}, "Method Flags"={"IsDeprecated"=FALSE, "IsPrivate"=FALSE, "IsScripting"=FALSE, "IsNotInRun-Time"=FALSE}, "Divider"=FALSE}, {"Class Info"={"Unique ID string"="1", "Parent ID string"="", "Class Name (unlocalized)"="Application", "Class Name (localized)"="Application"}, "Method Info"={"Unique ID string"="95a", "Data name"="GetEnvModeDisplayName", "Short name (localized)"="GetEnvModeDisplayName", "Long name (localized)"="Get Environment Mode Display Name"}, "Method Flags"={"IsDeprecated"=FALSE, "IsPrivate"=FALSE, "IsScripting"=FALSE, "IsNotInRun-Time"=FALSE}, "Divider"=FALSE}, {"Class Info"={"Unique ID string"="1", "Parent ID string"="", "Class Name (unlocalized)"="Application", "Class Name (localized)"="Application"}, "Method Info"={"Unique ID string"="95b", "Data name"="ClearCompObjCache", "Short name (localized)"="ClearCompObjCache", "Long name (localized)"="Clear Compiled Object Cache"}, "Method Flags"={"IsDeprecated"=FALSE, "IsPrivate"=FALSE, "IsScripting"=FALSE, "IsNotInRun-Time"=TRUE}, "Divider"=FALSE}, {"Class Info"={"Unique ID string"="1", "Parent ID string"="", "Class Name (unlocalized)"="Application", "Class Name (localized)"="Application"}, "Method Info"={"Unique ID string"="95c", "Data name"="Packed Library.Get Exported File List", "Short name (localized)"="Packed Library.Get Exported File List", "Long name (localized)"="Packed Library:Get Exported File List"}, "Method Flags"={"IsDeprecated"=FALSE, "IsPrivate"=TRUE, "IsScripting"=FALSE, "IsNotInRun-Time"=FALSE}, "Divider"=FALSE}, {"Class Info"={"Unique ID string"="1", "Parent ID string"="", "Class Name (unlocalized)"="Application", "Class Name (localized)"="Application"}, "Method Info"={"Unique ID string"="95d", "Data name"="Library.IsOpenedInAnyContext", "Short name (localized)"="Library.IsOpenedInAnyContext", "Long name (localized)"="Library:Is Opened In Any Context"}, "Method Flags"={"IsDeprecated"=FALSE, "IsPrivate"=TRUE, "IsScripting"=FALSE, "IsNotInRun-Time"=TRUE}, "Divider"=FALSE}, {"Class Info"={"Unique ID string"="1", "Parent ID string"="", "Class Name (unlocalized)"="Application", "Class Name (localized)"="Application"}, "Method Info"={"Unique ID string"="95e", "Data name"="Compile App Context", "Short name (localized)"="Compile App Context", "Long name (localized)"="Compiler:Compile App Context"}, "Method Flags"={"IsDeprecated"=FALSE, "IsPrivate"=TRUE, "IsScripting"=FALSE, "IsNotInRun-Time"=FALSE}, "Divider"=FALSE}, {"Class Info"={"Unique ID string"="1", "Parent ID string"="", "Class Name (unlocalized)"="Application", "Class Name (localized)"="Application"}, "Method Info"={"Unique ID string"="95f", "Data name"="Packed Library.Enable Caching", "Short name (localized)"="Packed Library.Enable Caching", "Long name (localized)"="Packed Library:Enable Caching"}, "Method Flags"={"IsDeprecated"=FALSE, "IsPrivate"=TRUE, "IsScripting"=FALSE, "IsNotInRun-Time"=FALSE}, "Divider"=FALSE}, {"Class Info"={"Unique ID string"="1", "Parent ID string"="", "Class Name (unlocalized)"="Application", "Class Name (localized)"="Application"}, "Method Info"={"Unique ID string"="960", "Data name"="Simulation.GetParamOffsets", "Short name (localized)"="Simulation.GetParamOffsets", "Long name (localized)"="Simulation:Get Parameter Offsets"}, "Method Flags"={"IsDeprecated"=FALSE, "IsPrivate"=TRUE, "IsScripting"=FALSE, "IsNotInRun-Time"=FALSE}, "Divider"=FALSE}, {"Class Info"={"Unique ID string"="1", "Parent ID string"="", "Class Name (unlocalized)"="Application", "Class Name (localized)"="Application"}, "Method Info"={"Unique ID string"="961", "Data name"="LVRT.Get LibP Sigs", "Short name (localized)"="LVRT.Get LibP Sigs", "Long name (localized)"="LVRT:Get Packed Library Signatures"}, "Method Flags"={"IsDeprecated"=FALSE, "IsPrivate"=TRUE, "IsScripting"=FALSE, "IsNotInRun-Time"=TRUE}, "Divider"=FALSE}, {"Class Info"={"Unique ID string"="1", "Parent ID string"="", "Class Name (unlocalized)"="Application", "Class Name (localized)"="Application"}, "Method Info"={"Unique ID string"="962", "Data name"="Open.VI Without Refees", "Short name (localized)"="Open.VI Without Refees", "Long name (localized)"="Open:VI Without Refees"}, "Method Flags"={"IsDeprecated"=FALSE, "IsPrivate"=TRUE, "IsScripting"=FALSE, "IsNotInRun-Time"=FALSE}, "Divider"=FALSE}, {"Class Info"={"Unique ID string"="1", "Parent ID string"="", "Class Name (unlocalized)"="Application", "Class Name (localized)"="Application"}, "Method Info"={"Unique ID string"="963", "Data name"="Build.Object Cache", "Short name (localized)"="Build.Object Cache", "Long name (localized)"="Build:Object Cache"}, "Method Flags"={"IsDeprecated"=FALSE, "IsPrivate"=TRUE, "IsScripting"=FALSE, "IsNotInRun-Time"=TRUE}, "Divider"=FALSE}, {"Class Info"={"Unique ID string"="1", "Parent ID string"="", "Class Name (unlocalized)"="Application", "Class Name (localized)"="Application"}, "Method Info"={"Unique ID string"="964", "Data name"="Install Adjacent Cache", "Short name (localized)"="Install Adjacent Cache", "Long name (localized)"="Install Adjacent Cache"}, "Method Flags"={"IsDeprecated"=FALSE, "IsPrivate"=TRUE, "IsScripting"=FALSE, "IsNotInRun-Time"=TRUE}, "Divider"=FALSE}, {"Class Info"={"Unique ID string"="1", "Parent ID string"="", "Class Name (unlocalized)"="Application", "Class Name (localized)"="Application"}, "Method Info"={"Unique ID string"="965", "Data name"="Get Palette Statistics", "Short name (localized)"="Get Palette Statistics", "Long name (localized)"="Palettes:Get Palette Statistics"}, "Method Flags"={"IsDeprecated"=FALSE, "IsPrivate"=TRUE, "IsScripting"=FALSE, "IsNotInRun-Time"=TRUE}, "Divider"=FALSE}, {"Class Info"={"Unique ID string"="1", "Parent ID string"="", "Class Name (unlocalized)"="Application", "Class Name (localized)"="Application"}, "Method Info"={"Unique ID string"="966", "Data name"="Force Finsh Load All Palettes", "Short name (localized)"="Force Finsh Load All Palettes", "Long name (localized)"="Palettes:Force Finsh Load All Palettes"}, "Method Flags"={"IsDeprecated"=FALSE, "IsPrivate"=TRUE, "IsScripting"=FALSE, "IsNotInRun-Time"=TRUE}, "Divider"=FALSE}, {"Class Info"={"Unique ID string"="1", "Parent ID string"="", "Class Name (unlocalized)"="Application", "Class Name (localized)"="Application"}, "Method Info"={"Unique ID string"="967", "Data name"="FlushArcCaching", "Short name (localized)"="FlushArcCaching", "Long name (localized)"="Flush Archive Caching"}, "Method Flags"={"IsDeprecated"=FALSE, "IsPrivate"=TRUE, "IsScripting"=TRUE, "IsNotInRun-Time"=FALSE}, "Divider"=FALSE}, {"Class Info"={"Unique ID string"="1", "Parent ID string"="", "Class Name (unlocalized)"="Application", "Class Name (localized)"="Application"}, "Method Info"={"Unique ID string"="968", "Data name"="ClearSpecCompObjCache", "Short name (localized)"="ClearSpecCompObjCache", "Long name (localized)"="Clear Specific Compiled Object Cache"}, "Method Flags"={"IsDeprecated"=FALSE, "IsPrivate"=TRUE, "IsScripting"=FALSE, "IsNotInRun-Time"=TRUE}, "Divider"=FALSE}, {"Class Info"={"Unique ID string"="1", "Parent ID string"="", "Class Name (unlocalized)"="Application", "Class Name (localized)"="Application"}, "Method Info"={"Unique ID string"="969", "Data name"="Restart", "Short name (localized)"="Restart", "Long name (localized)"="Restart"}, "Method Flags"={"IsDeprecated"=FALSE, "IsPrivate"=FALSE, "IsScripting"=FALSE, "IsNotInRun-Time"=FALSE}, "Divider"=FALSE}, {"Class Info"={"Unique ID string"="1", "Parent ID string"="", "Class Name (unlocalized)"="Application", "Class Name (localized)"="Application"}, "Method Info"={"Unique ID string"="970", "Data name"="Get Compiled Object File", "Short name (localized)"="Get Compiled Object File", "Long name (localized)"="GetCompiledObjectFile"}, "Method Flags"={"IsDeprecated"=FALSE, 
